vi "MainNR.vi"(10 "RQMHStartup":refnum<class "RQMHStartup.lvclass">, 11 "Header in":refnum<class "Header.lvclass">) -> ()   [LabVIEW 2024, in "Header.lvclass"]
uses:
  Header.lvclass
  RQMHCore/Startup/RQMHStartup.lvclass
  RQMHCore/ModQueue/RQMHMessageQueue.lvclass/RQMHMessageQueue.ctl
  RQMHCore/ModuleCore/InitialiseReplyArgs.ctl
  RQMHCore/ModuleCore/RQMHModule.lvclass/RQMHModule.ctl
  Do Something ReplyArgs.ctl
  Do Something Args.ctl
  RQMHCore/ModuleCore/Read ModuleName.vi
  RQMHCore/ModuleCore/Read External Start.vi
  RQMHCore/ModQueue/Delacor_lib_QMH_Enqueue Message (Single).vi
  RQMHCore/ModQueue/RQMHMessageQueue.lvclass
  RQMHCore/ModuleCore/RQMHModule.lvclass
  RQMHCore/Shared/RQMHShared.lvlib
panel:
  out "error out":errorcluster
  in  "Engineering":bool
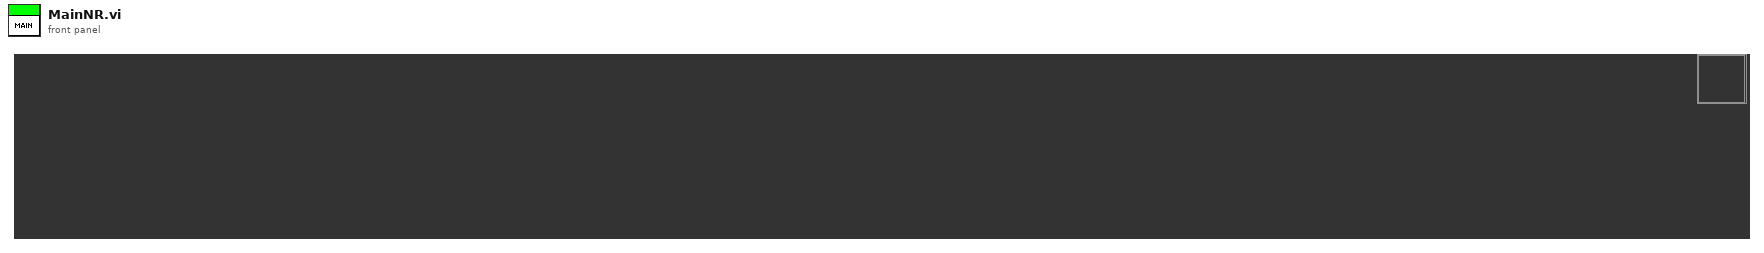
[diagram p1: front panel]
types:
  T1 = typedef "Header.lvclass/Request Events--cluster.ctl" = cluster{"Do Something":refnum<user-event>, "Add Menu Item":refnum<user-event>}
  T2 = cluster{"Stop Module":refnum<user-event>, "Requests":T1}
  T3 = enum32{"Invalid", "Standard", "Closed", "Hidden", "Minimized", "Maximized"}
  T4 = typedef "RQMHModule.lvclass/InitialiseReplyArgs.ctl" = cluster{"Did Init?":bool}
  T5 = typedef "Header.lvclass/Do Something Args.ctl" = cluster{"Msg":string}
  T6 = typedef "Header.lvclass/Do Something ReplyArgs.ctl" = cluster{"Value":dbl, "Boolean":bool}
  T7 = typedef "RQMHModule.lvclass/Reply.ctl" = cluster{"Expects Reply":bool, "Reply":refnum<notifier>}
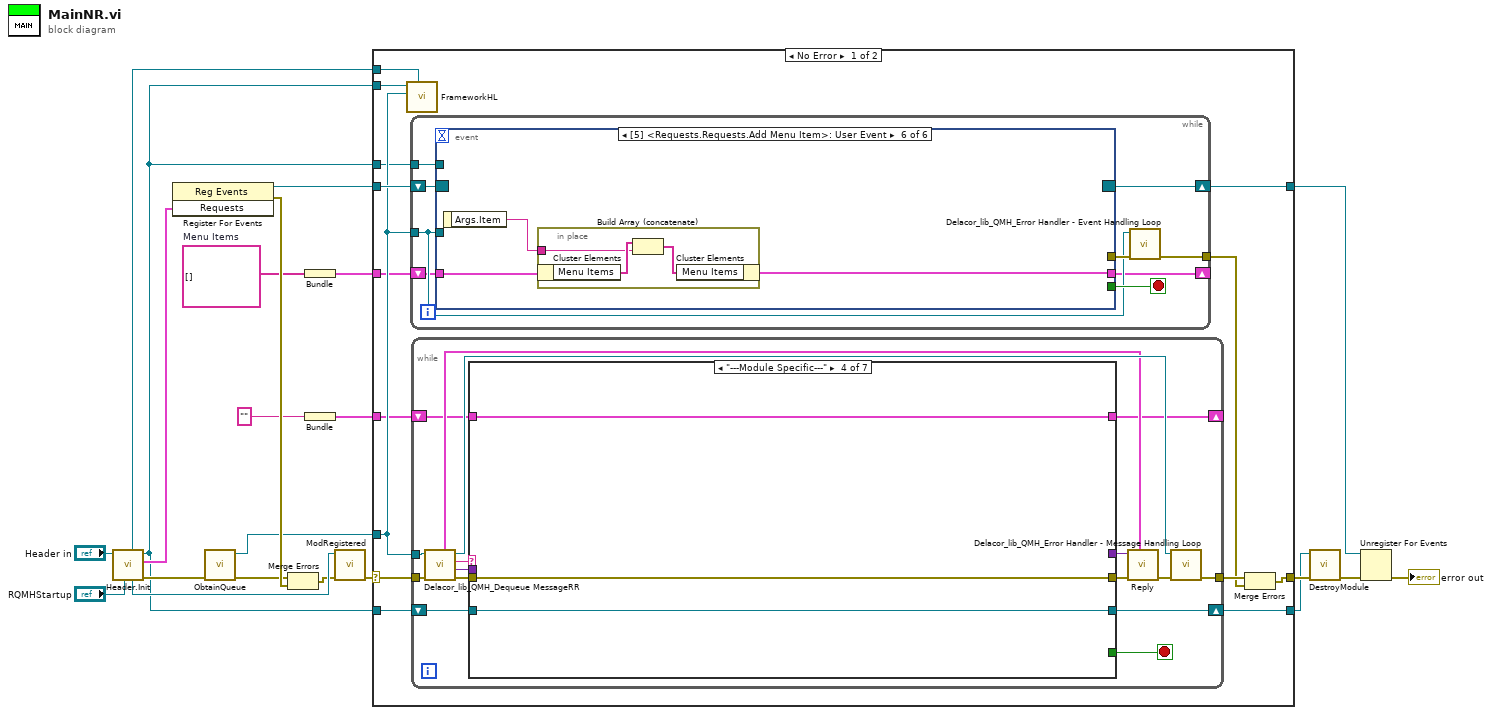
[diagram p0: block diagram]
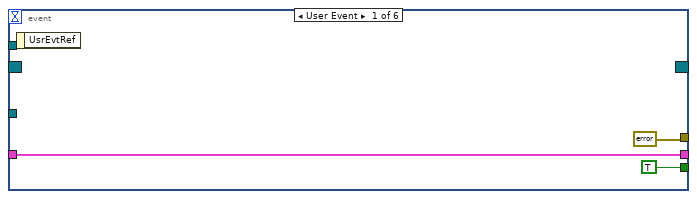
[diagram p2: hidden frame]
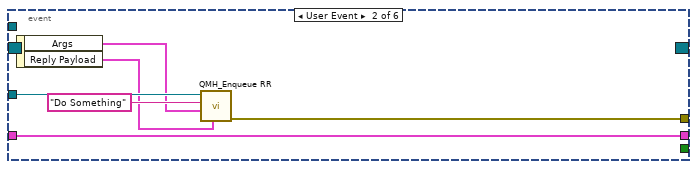
[diagram p3: hidden frame]
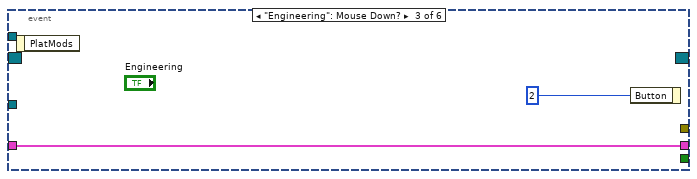
[diagram p4: hidden frame]
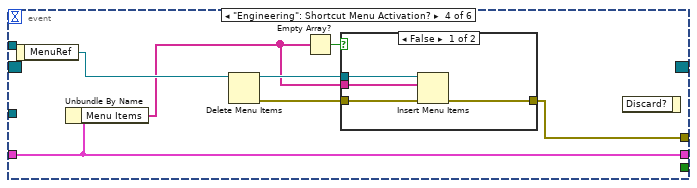
[diagram p5: hidden frame]
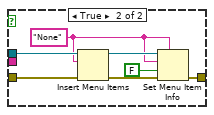
[diagram p6: hidden frame]
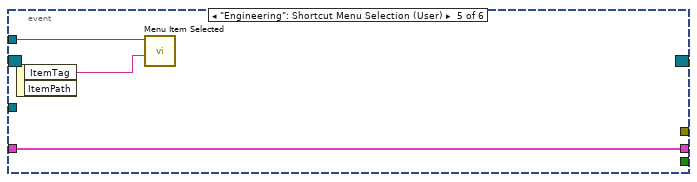
[diagram p7: hidden frame]
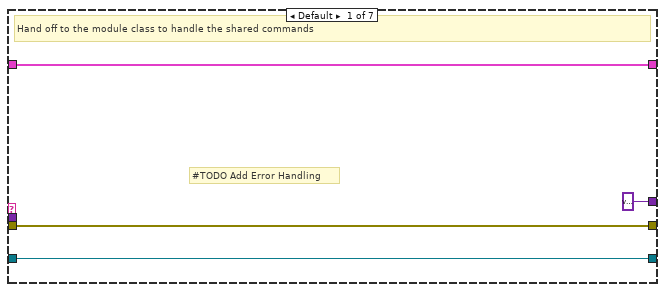
[diagram p8: hidden frame]
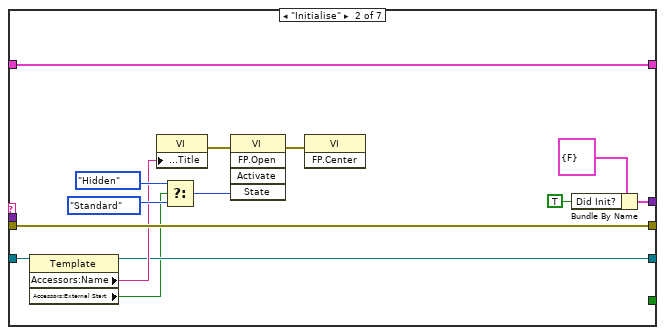
[diagram p9: hidden frame]
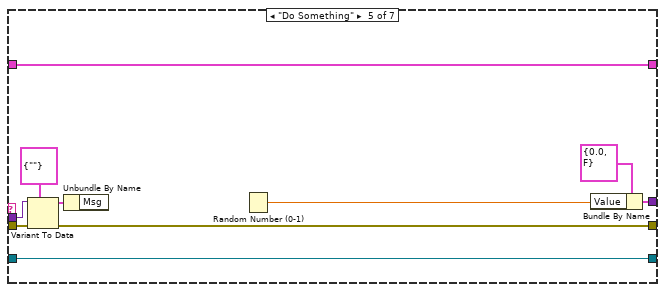
[diagram p11: hidden frame]
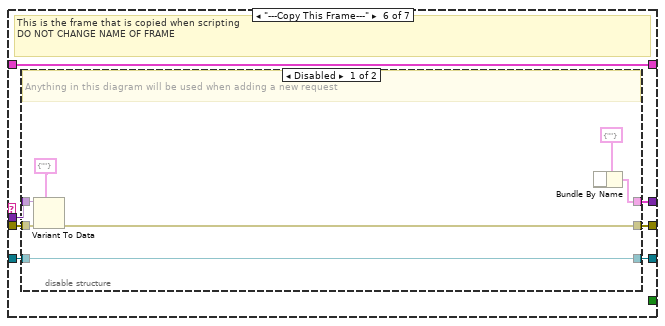
[diagram p12: hidden frame]
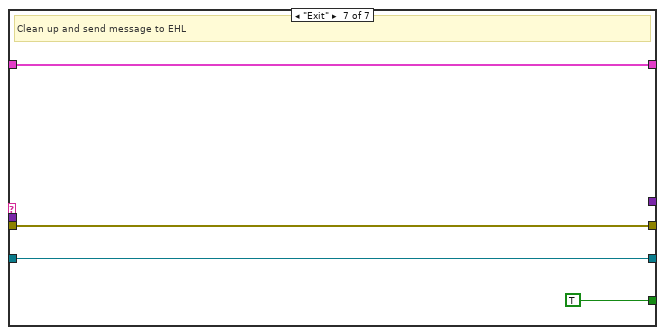
[diagram p14: hidden frame]
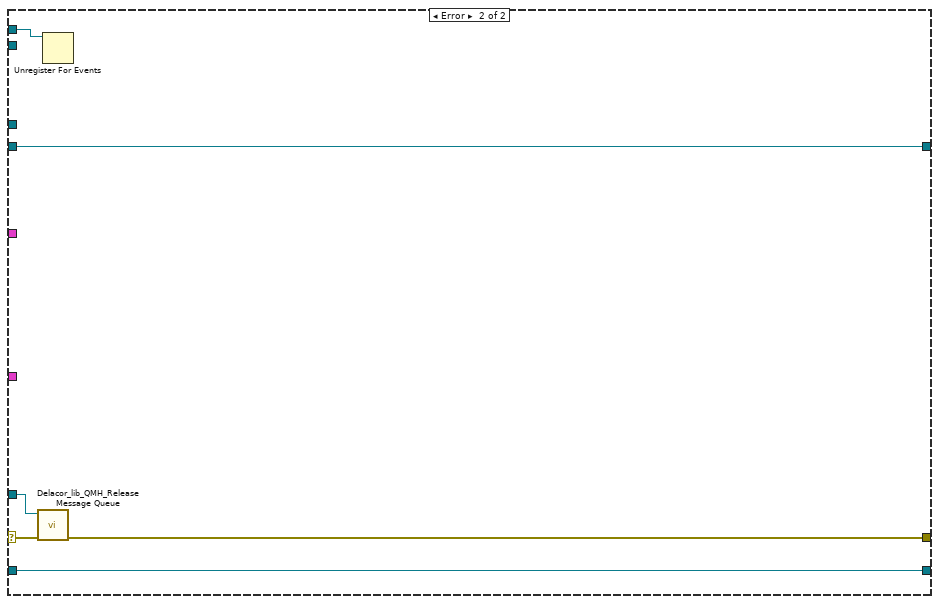
[diagram p15: hidden frame]
diagram:
  w4 = string[] []  # Menu Items
  n1 = call "Header.Init.vi"("JQMHStartup in"="RQMHStartup", "NewTemplate in"="Header in") -> ("error out"=w15:errorcluster, "Requests"=w6:T2, "NewTemplate out"=w1:refnum<class "Header.lvclass">, "JQMHStartup out"=w13:refnum<class "RQMHStartup.lvclass">, "StandardRequests"=w9:refnum<event-registration>)  [unwired: 3 in, 2 out]
  n2 = register-events(w6) -> (reference out=w8:refnum<event-registration>, error out=w22:errorcluster)  [unwired: 2 in]
  n3 = call "ObtainQueue.vi"("error in"=w15) -> ("error out"=w14:errorcluster, "Message Queue"=w10:refnum<class "RQMHMessageQueue.lvclass">)  [unwired: 9 in]
  n4 = Merge Errors(w14, w22) -> (w11:errorcluster)
  n5 = Bundle("Menu Items"=w4) -> (w3:cluster{"Menu Items":string[]})  [unwired: 1 in]
  n6 = Bundle("") -> (w5:cluster{string})  [unwired: 1 in]
  n7 = call "ModRegistered.vi"("error in (no error)"=w11, "JQMHStartup in"=w13) -> ("error out"=w12:errorcluster)  [unwired: 9 in]
  n8 = case "RQMH_MAIN" shown="No Error" w12 {
    selector: w12 -> [w33 w157]
    tunnel: w1 -> [w36 w156]
    tunnel: [w35 w159] -> w21
    tunnel: w8 -> [w34 w159]
    tunnel: w10 -> [w27 w158]
    tunnel: [w32 w156] -> w7
    tunnel: [w29 w155] -> w18
    tunnel: w1 -> [w28 _]
    tunnel: w9 -> [w26 w154]
    tunnel: w5 -> [w25 _]
    tunnel: w3 -> [w24 _]
    tunnel: w1 -> [w23 _]
    frame No Error {
      n9 = call-dynamic "FrameworkHL.vi"("StandardRequests"=w26, "Message Queue"=w27, "JQMHModule in"=w28) -> ()  [unwired: 9 in]
      n10 = while {
        shift-right: [w45] -> w35
        shift-left: w34 -> [w40]
        tunnel: w27 -> [w41]
        tunnel: [w42] -> w30
        shift-right: [w38] -> _
        shift-left: w24 -> [w39]
        tunnel: w23 -> [w37]
        stop <- w44 stop-if-true
        n11 = event "RQMH_EVENT_MAIN" shown="[5] <Requests.Requests.Add Menu Item>: User Event" {
          selector: w40 -> [_ _ _ _ _ _]
          dyn-events: [_ _ _ _ _ _] -> w45
          timeout: _ -> [_ _ _ _ _ _]
          tunnel: [TRUE _ _ _ _ _] -> w44
          tunnel: w41 -> [_ w54 _ _ _ _]
          tunnel: [errorcluster {"status"=FALSE, "code"=0, "source"=""} ("error out") w51 _ w57 _ _] -> w43
          tunnel: w39 -> [w46 w49 w55 w59 w77 w80]
          tunnel: [w46 w49 w55 w59 w77 w79] -> w38
          tunnel: w37 -> [_ _ _ _ w76 _]
          event User Event {
            n12 = event-data() -> ()  [unwired: 1 in, 1 out]
          }
          event User Event {
            n13 = event-data() -> ("Args"=w52:T5, "Reply Payload"=w50:T7)  [unwired: 1 in]
            n14 = call "QMH_Enqueue RR.vi"("Reply"=w50, "Message Data"=w52, "Message"="Do Something", "Message Queue in"=w54) -> ("error out"=w51:errorcluster)  [unwired: 6 in, 1 out]
          }
          event "Engineering": Mouse Down? {
            n15 = event-data() -> ()  [unwired: 1 in, 1 out]
            n16 = event-data("Button"=u16 2) -> ()  [unwired: 1 in, 1 out]
          }
          event "Engineering": Shortcut Menu Activation? {
            n17 = event-data() -> ("MenuRef"=w60:refnum<k9>)  [unwired: 1 in]
            n18 = Unbundle By Name(w59) -> ("Menu Items"=w58:string[])
            n19 = Delete Menu Items(9:w60) -> (0:w62:errorcluster, 3:w63:refnum<k9>)  [unwired: 3 in]
            n20 = Empty Array?(array=w58) -> (empty?=w61:bool)
            n21 = case shown="False" w61 {
              tunnel: w63 -> [w67 w74]
              tunnel: w62 -> [w66 w73]
              tunnel: w58 -> [w64 _]
              tunnel: [w65 w70] -> w57
              frame False {
                n22 = Insert Menu Items(6:w66, 8:w64, 9:w67) -> (0:w65:errorcluster)  [unwired: 3 in, 2 out]
              }
              frame True {
                w68 = "None"
                n23 = Insert Menu Items(6:w73, 8:w68, 9:w74) -> (0:w71:errorcluster, 3:w72:refnum<k9>)  [unwired: 3 in, 1 out]
                n24 = Set Menu Item Info(7:w68, 8:w71, 9:FALSE ("enabled"), 10:w68, 11:w72) -> (0:w70:errorcluster)  [unwired: 2 in, 1 out]
              }
            }
            n25 = event-data() -> ()  [unwired: 2 in, 1 out]
          }
          event "Engineering": Shortcut Menu Selection (User) {
            n26 = event-data() -> ("ItemTag"=w75:string)  [unwired: 1 in, 1 out]
            n27 = call "Menu Item Selected.vi"("Menu Item"=w75, "module in"=w76) -> ()  [unwired: 8 in, 2 out]
          }
          event User Event {
            n28 = event-data() -> ("Args.Item"=w78:string)  [unwired: 1 in]
            n29 = in-place {
              in-place-border: w78 -> [w81]
              n30 = in-place-cluster #1(w80) -> ("Menu Items"=w83:string[])
              n31 = Build Array (concatenate)(w83, w81) -> (w82:string[])
              n32 = in-place-cluster #1("Menu Items"=w82) -> (w79:cluster{"Menu Items":string[]})
            }
          }
        }
        n33 = call-dynamic "Delacor_lib_QMH_Error Handler - Event Handling Loop.vi"("error in"=w43, "Message Queue in"=w41) -> ("dup error in"=w42:errorcluster)  [unwired: 8 in, 1 out]
      }
      n34 = while {
        tunnel: w27 -> [w94]
        tunnel: w33 -> [w93]
        shift-right: [w96] -> w32
        shift-left: w36 -> [w97]
        tunnel: [w95] -> w31
        shift-right: [w85] -> _
        shift-left: w25 -> [w84]
        stop <- w99 stop-if-true
        n35 = call-dynamic "Delacor_lib_QMH_Dequeue MessageRR.vi"("error in"=w93, "Message Queue in"=w94) -> ("error out"=w92:errorcluster, "Message Data"=w90:variant, "Message"=w91:string, "Message Queue out"=w98:refnum<class "RQMHMessageQueue.lvclass">, "Reply"=w86:T7)  [unwired: 5 in]
        n36 = case "RQMH_MESSAGE_CASES" shown="\"---Module Specific---\"" w91 {
          tunnel: [_ _ _ _ _ _ TRUE] -> w99
          tunnel: w97 -> [w102 w106 w119 w122 w133 w138 w152]
          tunnel: w90 -> [_ _ _ _ w129 w136 _]
          tunnel: w92 -> [w103 w117 w120 w123 w128 w140 w151]
          tunnel: [w103 w117 w120 w123 w127 w139 w151] -> w89
          tunnel: [w102 w107 w119 w122 w133 w137 w152] -> w96
          tunnel: [variant w116 _ _ w132 w135 _] -> w87
          tunnel: [w100 w104 w118 w121 w124 w134 w150] -> w85
          tunnel: w84 -> [w100 w104 w118 w121 w124 w134 w150]
          frame Default {
            # "#TODO Add Error Handling"
            # "Hand off to the module class to handle the shared commands"
          }
          frame "Initialise" {
            n37 = property class="Template"(reference=w106) -> (reference out=w107:refnum<class "Header.lvclass">, "Accessors:Name"=w108:string, "Accessors:External Start"=w105:bool)  [unwired: 1 in, 1 out]
            n38 = property on="Property Node" class="VI"("Front Panel.Title"=w108) -> (error out=w114:errorcluster)  [unwired: 2 in, 1 out]
            n39 = Select(t=T3."Hidden" ("State"), s=w105, f=T3."Standard" ("State")) -> (s? t:f=w110:T3)
            n40 = invoke on="Invoke Node" class="VI" method="FP.Open"(error in=w114, "State"=w110) -> (error out=w113:errorcluster)  [unwired: 3 in, 4 out]
            n41 = invoke on="Invoke Node" class="VI" method="FP.Center"(error in=w113) -> ()  [unwired: 2 in, 3 out]
            n42 = Bundle By Name(cluster=T4 {"Did Init?"=FALSE} ("Args"), "Did Init?"=TRUE) -> (w116:T4)
          }
          frame "---Internal---" {
          }
          frame "---Module Specific---" {
          }
          frame "Do Something" {
            n43 = Variant To Data(error in=w128, type=T5 {"Msg"=""} ("Do Something Args"), Variant=w129) -> (data=w125:T5, error out=w127:errorcluster)
            n44 = Unbundle By Name(w125) -> ()  [unwired: 1 out]
            n45 = Random Number (0-1)() -> (number: 0 to 1=w130:dbl)
            n46 = Bundle By Name(cluster=T6 {"Value"=0.0, "Boolean"=FALSE}, "Value"=w130) -> (w132:T6)
          }
          frame "---Copy This Frame---" {
            # "This is the frame that is copied when scripting\nDO NOT CHANGE NAME OF FRAME"
            n47 = disable-structure shown="Disabled" {
              disable-tunnel: w140 -> [w144 w149]
              disable-tunnel: [w145 w149] -> w139
              disable-tunnel: w138 -> [w147 w148]
              disable-tunnel: [w147 w148] -> w137
              disable-tunnel: w136 -> [w146 _]
              disable-tunnel: [w142 _] -> w135
              frame Disabled {
                # "Anything in this diagram will be used when adding a new request"
                n48 = Variant To Data(error in=w144, type=cluster{string} {""} ("RQMH_MHL_MSG_PL"), Variant=w146) -> (error out=w145:errorcluster)  [unwired: 1 out]
                n49 = Bundle By Name(cluster=cluster{string} {""} ("RQMH_MHL_REPLY_PL")) -> (w142:cluster{string})  [unwired: 1 in]
              }
              frame Enabled {
              }
            }
          }
          frame "Exit" {
            # "Clean up and send message to EHL"
          }
        }
        n50 = call "Reply.vi"("Reply"=w86, "error in (no error)"=w89, "ReplyPayload"=w87) -> ("error out"=w88:errorcluster)  [unwired: 8 in]
        n51 = call-dynamic "Delacor_lib_QMH_Error Handler - Message Handling Loop.vi"("error in"=w88, "Message Queue in"=w98) -> ("dup error in"=w95:errorcluster)  [unwired: 8 in, 1 out]
      }
      n52 = Merge Errors(w31, w30) -> (w29:errorcluster)
    }
    frame Error {
      n53 = call-dynamic "Delacor_lib_QMH_Release Message Queue.vi"("error in"=w157, "Message Queue"=w158) -> ("error out"=w155:errorcluster)  [unwired: 9 in]
      n54 = Unregister For Events(event registration refnum=w154) -> ()  [unwired: 1 in, 1 out]
    }
  }
  n55 = call "DestroyModule.vi"("error in (no error)"=w18, "JQMHModule in"=w7) -> ("error out"=w20:errorcluster)  [unwired: 9 in]
  n56 = Unregister For Events(event registration refnum=w21, error in=w20) -> (error out=→"error out":errorcluster)
